vi "read test param.vi"(8 "error in (no error)":errorcluster, 10 "File Path":path, 11 "Solenoid in":refnum<class "Solenoid.lvclass">) -> (0 "error out":errorcluster, 3 "Solenoid out":refnum<class "Solenoid.lvclass">)   [LabVIEW 2025, in "Solenoid.lvclass"]
uses:
  Solenoid.lvclass
  Solenoid.lvclass/Solenoid.ctl
  2462b18c-1aa2-4af3-ba69-5179fb670ccf.vi
  <vilib>/JDP Science/JSONtext/JSON text to Variant.vi
  <vilib>/JDP Science/JSONtext/LVClass Serializer/JSONtext LVClass Serializer.lvclass
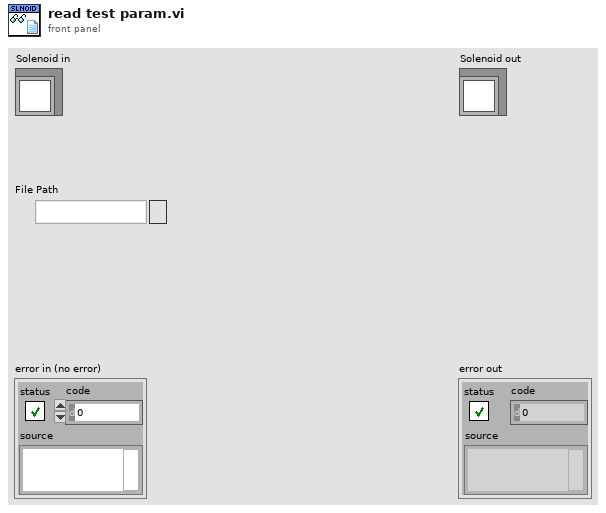
[diagram p1: front panel]
types:
  T1 = typedef "json cluster.ctl" = cluster{"Electrical_Properties":cluster{"V_max":dbl, "I_max":dbl}, "Wear_in":cluster{"V":dbl, "I":dbl, "Cycles":dbl, "On_Time_ms":dbl, "Off_Time_ms":dbl}, "Drop_out":cluster{"V":dbl, "I":dbl, "V_reduced":dbl, "V_perturb":dbl, "Plunger_Threshold":dbl, "V_MIN":dbl}, "ORT":cluster{"V":dbl, "I":dbl, "ORT_MAX_ms":dbl}, "CRT":cluster{"V":dbl, "I":dbl, "ORT_MAX_ms":dbl}, "Pull_in":cluster{"V":dbl, "I":dbl, "V_increased":dbl, "V_perturb":dbl, "Plunger_Threshold":dbl, "V_MAX":dbl}, "Coil_Resistance":cluster{"V":dbl, "I":dbl, "R_MAX":dbl, "R_MIN":dbl}}
  T2 = cluster{"V":dbl, "I":dbl, "Cycles":dbl, "On_Time_ms":dbl, "Off_Time_ms":dbl}
  T3 = cluster{"V":dbl, "I":dbl, "V_reduced":dbl, "V_perturb":dbl, "Plunger_Threshold":dbl, "V_MIN":dbl}
  T4 = cluster{"V":dbl, "I":dbl, "V_increased":dbl, "V_perturb":dbl, "Plunger_Threshold":dbl, "V_MAX":dbl}
  T5 = cluster{"V":dbl, "I":dbl, "R_MAX":dbl, "R_MIN":dbl}
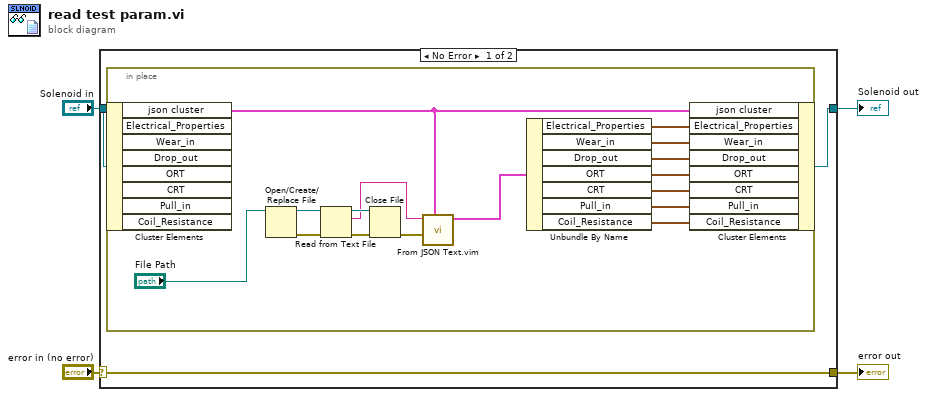
[diagram p0: block diagram]
diagram:
  n1 = case shown="No Error" "error in (no error)" {
    selector: "error in (no error)" -> [w7 w25]
    tunnel: [w7 w25] -> w3
    tunnel: [w6 w24] -> w1
    tunnel: "Solenoid in" -> [w5 w24]
    frame No Error {
      n2 = in-place {
        n3 = in-place-cluster #1(w5) -> ("json cluster"=w11:T1)  [unwired: 7 out]
        n4 = Open/Create/Replace File(file path (use dialog)="File Path") -> (refnum out=w23:refnum<file>, error out=w22:errorcluster)  [unwired: 5 in, 1 out]
        n5 = Read from Text File(file (use dialog)=w23, error in=w22) -> (refnum out=w20:refnum<file>, text=w19:string, error out=w21:errorcluster)  [unwired: 2 in, 1 out]
        n6 = Close File(refnum=w20, error in=w21) -> (error out=w18:errorcluster)  [unwired: 1 out]
        n7 = call "From JSON Text.vim"("Data Type and Default Value"=w11, "error in (no error)"=w18, "JSON"=w19) -> ("Data out"=w10:T1)  [unwired: 7 in, 1 out]
        n8 = Unbundle By Name(w10) -> ("Electrical_Properties"=w17:cluster{"V_max":dbl, "I_max":dbl}, "Wear_in"=w16:T2, "Drop_out"=w15:T3, "ORT"=w14:cluster{"V":dbl, "I":dbl, "ORT_MAX_ms":dbl}, "CRT"=w13:cluster{"V":dbl, "I":dbl, "ORT_MAX_ms":dbl}, "Pull_in"=w12:T4, "Coil_Resistance"=w8:T5)
        n9 = in-place-cluster #1("json cluster"=w11, "Electrical_Properties"=w17, "Wear_in"=w16, "Drop_out"=w15, "ORT"=w14, "CRT"=w13, "Pull_in"=w12, "Coil_Resistance"=w8) -> (w6:refnum<class "Solenoid.lvclass">)
      }
    }
    frame Error {
    }
  }
  "error out" <- w3
  "Solenoid out" <- w1
